vi "Distance from Image Name.vi"(10 "Image Name":string) -> (2 "Distance (km)":dbl)   [LabVIEW 2024]
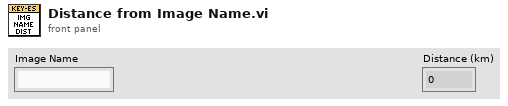
[diagram p1: front panel]
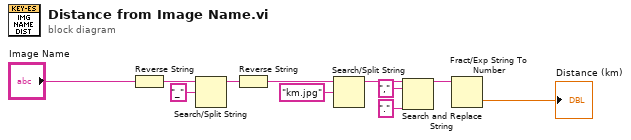
[diagram p0: block diagram]
diagram:
  n1 = Reverse String(1:"Image Name") -> (0:w11:string)
  n2 = Search/Split String(string=w11, search string/char (-)="_") -> (substring before match=w9:string)  [unwired: 1 in, 2 out]
  n3 = Reverse String(1:w9) -> (0:w8:string)
  n4 = Search/Split String(string=w8, search string/char (-)="km.jpg") -> (substring before match=w5:string)  [unwired: 1 in, 2 out]
  n5 = Search and Replace String(input string=w5, search string=",", replace string="." ("replace string (\"\")")) -> (result string=w2:string)  [unwired: 5 in, 3 out]
  n6 = Fract/Exp String To Number(string=w2) -> (number=→"Distance (km)":dbl)  [unwired: 3 in, 1 out]
